vi "Get Resource String by RID and LangIndex.vi"(8 "error in (no error)":errorcluster, 9 "LangIndex (0)":i32, 10 "RID":string, 11 "LangFile in":refnum<class "Resource Data.lvclass">) -> (0 "error out":errorcluster, 1 "Found?":bool, 2 "Translated Text (ASCII)":string, 3 "LangFile out":refnum<class "Resource Data.lvclass">)   [LabVIEW 2013, in "SET Project Data.lvlib" / "Resource Data.lvclass"]
uses:
  Resource Data.lvclass
  Resource Data.lvclass/Resource Data.ctl
  Read Languages.vi
  Lib/Unicode/SET_Unicode Tools.lvlib
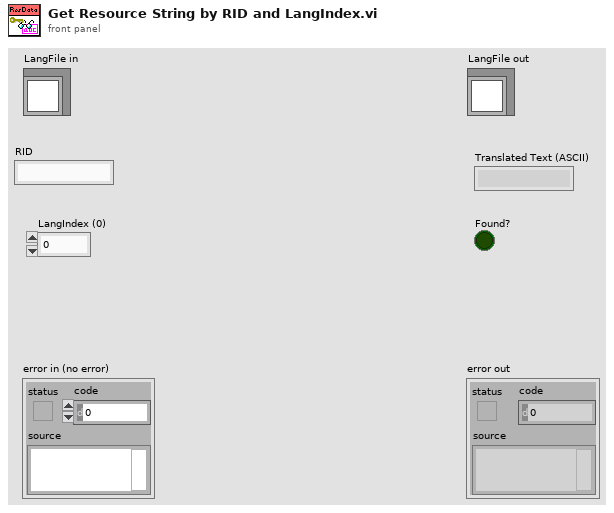
[diagram p1: front panel]
types:
  T1 = typedef "SET Project Data.lvlib/ProjFile_Resource Entry.ctl" = cluster{"RID":string, "Tag":string, "Strings [] (UTF-16)":string[], "Shared?":bool}
  T2 = typedef "SET Project Data.lvlib/ProjFile_Language Data.ctl" = cluster{"Tag":string, "Name":string, "Code Page":u16}
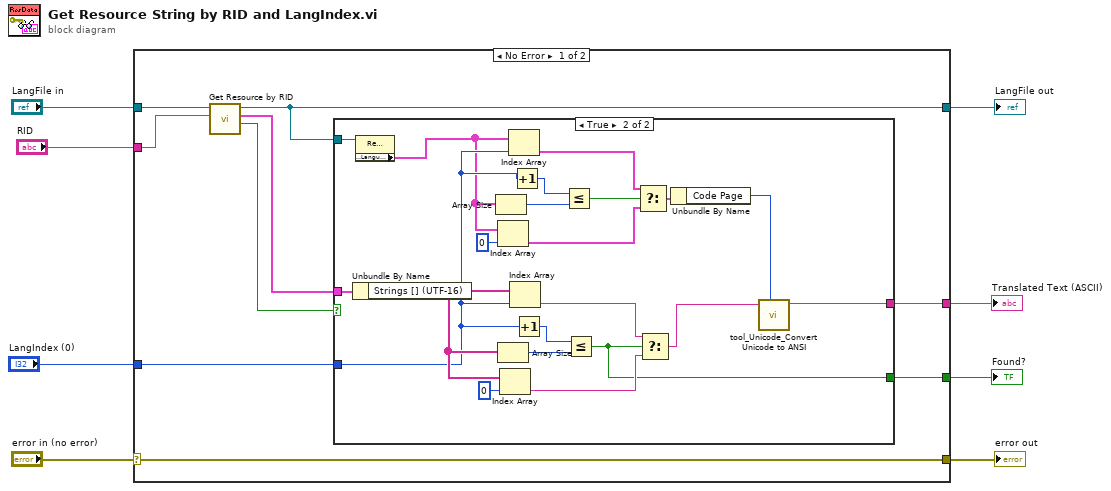
[diagram p0: block diagram]
diagram:
  n1 = case shown="No Error" "error in (no error)" {
    selector: "error in (no error)" -> [w17 w40]
    tunnel: [w17 w40] -> w7
    tunnel: [w14 w39] -> w5
    tunnel: "LangFile in" -> [w10 w39]
    tunnel: "RID" -> [w16 _]
    tunnel: "LangIndex (0)" -> [w9 _]
    tunnel: [w12 _] -> w2
    tunnel: [w11 _] -> w1
    frame No Error {
      n2 = call "Get Resource by RID.vi"("RID"=w16, "LangFile in"=w10) -> ("Found?"=w13:bool, "Resource"=w15:T1, "LangFile out"=w14:refnum<class "Resource Data.lvclass">)  [unwired: 5 in, 2 out]
      n3 = case shown="True" w13 {
        tunnel: w15 -> [_ w38]
        tunnel: w14 -> [_ w23]
        tunnel: w9 -> [_ w27]
        tunnel: [_ w20] -> w12
        tunnel: [_ w24] -> w11
        frame False {
        }
        frame True {
          n4 = Unbundle By Name(w38) -> ("Strings [] (UTF-16)"=w34:string[])
          n5 = property class="Resource Data.lvclass"(reference=w23) -> ("Properties:Languages []"=w22:T2[])  [unwired: 1 in, 2 out]
          n6 = Array Size(array=w22) -> (size(s)=w28:i32)
          n7 = Index Array(array=w22, index=0) -> (element=w31:T2)
          n8 = Array Size(array=w34) -> (size(s)=w37:i32)
          n9 = Index Array(array=w34, index=0) -> (element=w33:string)
          n10 = Index Array(array=w22, index=w27) -> (element=w25:T2)
          n11 = Index Array(array=w34, index=w27) -> (element=w32:string)
          n12 = Increment(x=w27) -> (x+1=w26:i32)
          n13 = Increment(x=w27) -> (x+1=w36:i32)
          n14 = Less Or Equal?(x=w26, y=w28) -> (x <= y?=w30:bool)
          n15 = Less Or Equal?(x=w36, y=w37) -> (x <= y?=w24:bool)
          n16 = Select(t=w25, s=w30, f=w31) -> (s? t:f=w19:T2)
          n17 = Select(t=w32, s=w24, f=w33) -> (s? t:f=w21:string)
          n18 = Unbundle By Name(w19) -> ("Code Page"=w18:u16)
          n19 = call "tool_Unicode_Convert Unicode to ANSI.vi"("Dest. Code Page"=w18, "WideChar (UTF16-LE)"=w21) -> ("MultiByteStr (ANSI)"=w20:string)  [unwired: 8 in, 1 out]
        }
      }
    }
    frame Error {
    }
  }
  "error out" <- w7
  "LangFile out" <- w5
  "Translated Text (ASCII)" <- w2
  "Found?" <- w1
